vi "Execute Previous Commands.vi"(8 "error in (no error)":errorcluster, 9 "length":i32, 10 "index":i32, 11 "Command Handler in":refnum<class "Command Handler.lvclass">) -> (0 "error out":errorcluster, 3 "Command Handler out":refnum<class "Command Handler.lvclass">)   [LabVIEW 2017, in "Command Handler.lvlib" / "Command Handler.lvclass"]
uses:
  Command Handler.lvclass
  Command Handler.lvclass/Command Handler.ctl
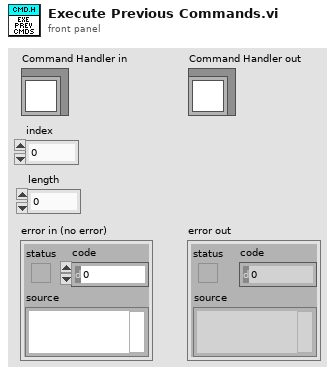
[diagram p1: front panel]
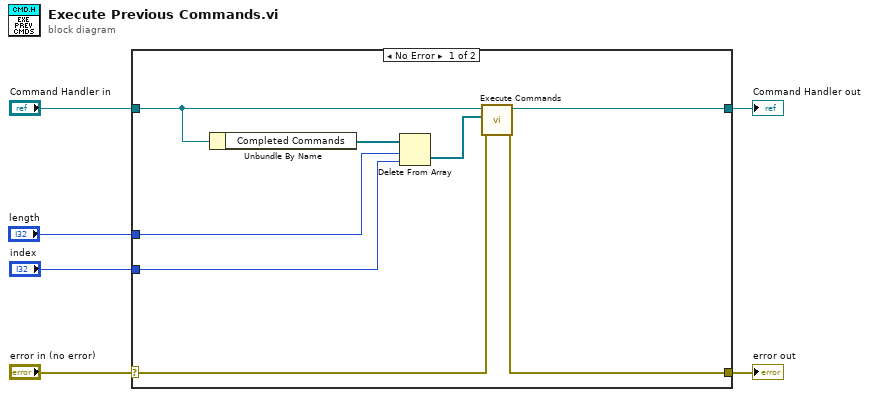
[diagram p0: block diagram]
diagram:
  n1 = case shown="No Error" "error in (no error)" {
    selector: "error in (no error)" -> [w11 w16]
    tunnel: [w10 w16] -> w5
    tunnel: [w12 w15] -> w3
    tunnel: "Command Handler in" -> [w13 w15]
    tunnel: "index" -> [w8 _]
    tunnel: "length" -> [w7 _]
    frame No Error {
      n2 = Unbundle By Name(w13) -> ("Completed Commands"=w14:refnum<class "Command.lvclass">[])
      n3 = Delete From Array(array=w14, length=w7, index=w8) -> (deleted portion=w9:refnum<class "Command.lvclass">[])  [unwired: 1 out]
      n4 = call-dynamic "Execute Commands.vi"("error in (no error)"=w11, "Command Array"=w9, "Command Handler in"=w13) -> ("error out"=w10:errorcluster, "Command Handler out"=w12:refnum<class "Command Handler.lvclass">)  [unwired: 7 in]
    }
    frame Error {
    }
  }
  "error out" <- w5
  "Command Handler out" <- w3
